vi "Pass Ref and Receive Data.vi"(7 "Enum State":T1=enum."Pass Data", 8 "error in (no error)":errorcluster, 10 "Data":T2={"Raw Data"=[], "Volt Channel"={"Index"=[], "Chl Name"=[], "Scale"=[], "Offset"=[], "Sample Rate"=100, "Device Name"="", "Channel"=""}}, 11 "Graph Manager in":refnum<class "Display Abstract.lvclass">) -> (0 "error out":errorcluster, 3 "Graph Manager out":refnum<class "Display Abstract.lvclass">)   [LabVIEW 2021, in "Display Abstract.lvclass"]
doc: "Do nothing."
uses:
  Display Abstract.lvclass
  Graph Data -- cluster.ctl
  Control/Volt Chl.ctl
  Pass Ref and Receive Data -- Enum.ctl
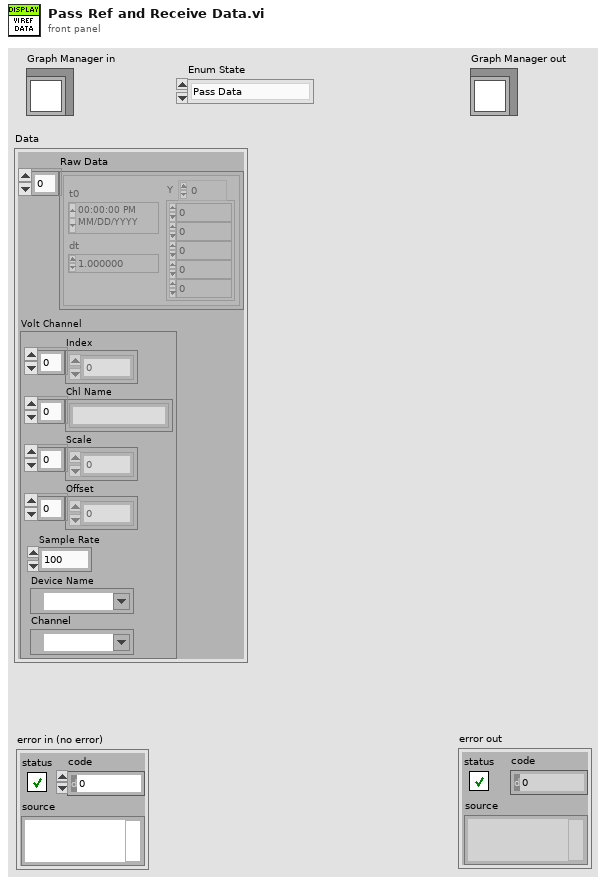
[diagram p1: front panel]
types:
  T1 = typedef "Pass Ref and Receive Data -- Enum.ctl" = enum16{"Initialize", "Pass Data"}
  T2 = typedef "Graph Data -- cluster.ctl" = cluster{"Raw Data":waveform(dbl)[], "Volt Channel":T3}
  T3 = typedef "Volt Chl.ctl" = cluster{"Index":i32[], "Chl Name":string[], "Scale":dbl[], "Offset":dbl[], "Sample Rate":i32, "Device Name":tag, "Channel":tag}
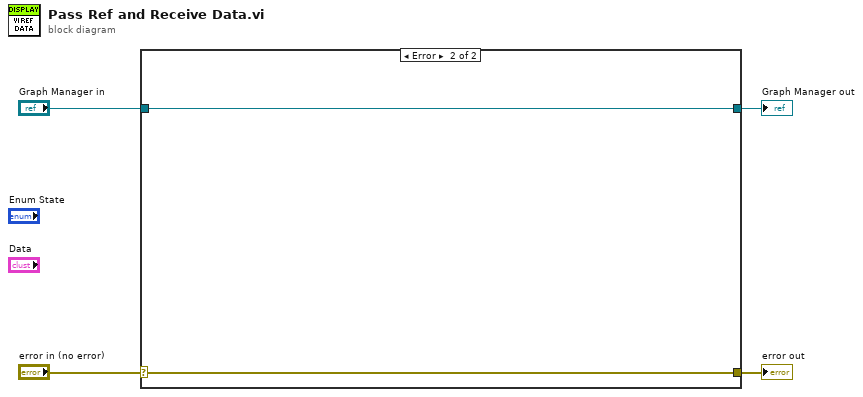
[diagram p0: block diagram]
diagram:
  n1 = case shown="Error" "error in (no error)" {
    selector: "error in (no error)" -> [w5 w8]
    tunnel: [w5 w8] -> w3
    tunnel: [w6 w7] -> w1
    tunnel: "Graph Manager in" -> [w6 w7]
    frame No Error {
      # "Wire the error cluster across even in the \"No Error\"\ncase so that warnings get propagated."
    }
    frame Error {
    }
  }
  "error out" <- w3
  "Graph Manager out" <- w1
